vi "Test File Log Provider.vi"() -> (1 "pass?":bool)   [LabVIEW 2019, in "ANODE Tests.lvlib"]
uses:
  ANODE Tests.lvlib
  ANODE/Utility API/Log Service/public/level.ctl
  34bea0a4-f80a-4efe-aaf4-9db1f3a8a041.vi
  4e885d52-342e-4d6f-86c2-bbc79adb3db9.vi
  901ffbec-7f76-4fda-a8b3-ab898965128c.vi
  31a8342b-9139-4bdf-bbc1-bb92f7179d80.vi
  c69379c1-06bc-43e8-abf1-6b6e803fbc34.vi
  7ff86ca6-88c0-4de2-a7d7-e18e6c48d840.vi
  f5e9308b-311a-4c07-9062-c62029aec88d.vi
  cd498dcc-2004-4e95-9cb1-3a88910e2f61.vi
  4bbd3971-874f-4069-8a4a-00f2533dc096.vi
  51edfdbb-9a3d-492a-8a02-2d0f54c6b824.vi
  8f198e5f-b4d0-4ca0-822a-d58fe651c8a2.vi
  ANODE/Util/Timestamp or now.vi
  ANODE/Utility API/File Log Provider/File Log Provider.lvclass
  C:/Users/Nicholas Folse/Documents/workspace/github-tauterra.llc/ANODE/ANODE/Utility API/Log Service/Log Service.lvclass
  ANODE/Utility API/Log Service/Log Service.lvclass
panel:
  out "log file text":string
  out "error out":errorcluster
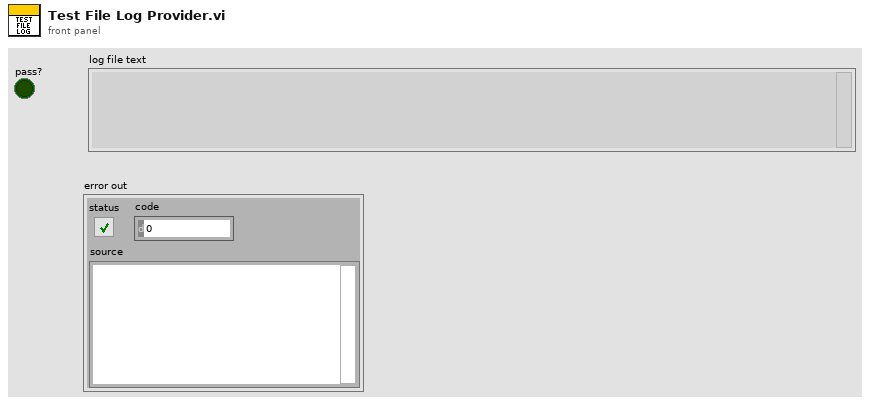
[diagram p1: front panel]
types:
  T1 = typedef "Utility API.lvlib/Log Service.lvclass/level.ctl" = u16
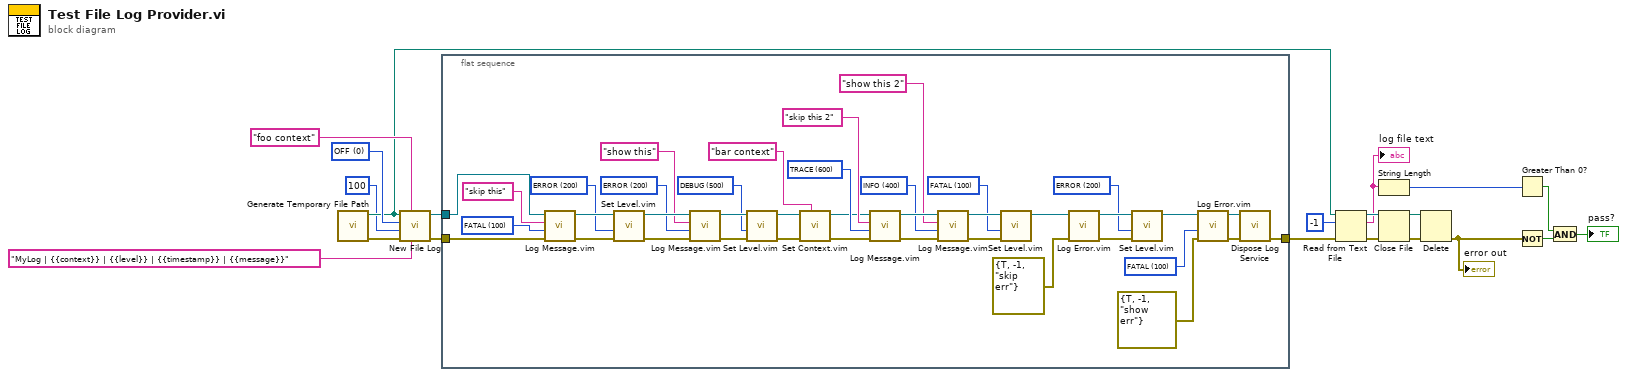
[diagram p0: block diagram]
diagram:
  w19 = T1 0 items=["OFF"=0, "FATAL"=100, "ERROR"=200, "WARN"=300, "INFO"=400, "DEBUG"=500, "TRACE"=600, "ALL"=65535] ("level")
  n1 = call <vilib>:"Generate Temporary File Path.vi"() -> ("error out"=w6:errorcluster, "Unique Temporary File Path"=w16:path)  [unwired: 10 in]
  n2 = call "New File Log.vi"("line format"="MyLog | {{context}} | {{level}} | {{timestamp}} | {{message}}", "context"="foo context", "error in (no error)"=w6, "write timeout (100ms)"=100, "level"=w19, "Path"=w16) -> ("error out"=w17:errorcluster, "File Log Provider out"=w18:refnum<data-value>)  [unwired: 4 in]
  n3 = flat-sequence {
    tunnel: w18 -> [w59]
    tunnel: w17 -> [w51]
    tunnel: [w23] -> w15
    frame #0 {
      w21 = T1 100 items=["OFF"=0, "FATAL"=100, "ERROR"=200, "WARN"=300, "INFO"=400, "DEBUG"=500, "TRACE"=600, "ALL"=65535] ("error level")
      w31 = T1 200 items=["OFF"=0, "FATAL"=100, "ERROR"=200, "WARN"=300, "INFO"=400, "DEBUG"=500, "TRACE"=600, "ALL"=65535] ("level")
      w36 = T1 100 items=["OFF"=0, "FATAL"=100, "ERROR"=200, "WARN"=300, "INFO"=400, "DEBUG"=500, "TRACE"=600, "ALL"=65535] ("level")
      w39 = T1 400 items=["OFF"=0, "FATAL"=100, "ERROR"=200, "WARN"=300, "INFO"=400, "DEBUG"=500, "TRACE"=600, "ALL"=65535] ("level")
      w43 = T1 600 items=["OFF"=0, "FATAL"=100, "ERROR"=200, "WARN"=300, "INFO"=400, "DEBUG"=500, "TRACE"=600, "ALL"=65535] ("level")
      w46 = T1 500 items=["OFF"=0, "FATAL"=100, "ERROR"=200, "WARN"=300, "INFO"=400, "DEBUG"=500, "TRACE"=600, "ALL"=65535] ("level")
      w52 = T1 200 items=["OFF"=0, "FATAL"=100, "ERROR"=200, "WARN"=300, "INFO"=400, "DEBUG"=500, "TRACE"=600, "ALL"=65535] ("level")
      w55 = T1 200 items=["OFF"=0, "FATAL"=100, "ERROR"=200, "WARN"=300, "INFO"=400, "DEBUG"=500, "TRACE"=600, "ALL"=65535] ("level")
      w58 = T1 100 items=["OFF"=0, "FATAL"=100, "ERROR"=200, "WARN"=300, "INFO"=400, "DEBUG"=500, "TRACE"=600, "ALL"=65535] ("level")
      n4 = call "Log Message.vim"("error in (no error)"=w51, "level"=w58, "message"="skip this", "Log Service in"=w59) -> ("error out"=w50:errorcluster, "Log Service out"=w56:refnum<data-value>)  [unwired: 6 in]
      n5 = call "Set Level.vim"("error in (no error)"=w50, "level"=w55, "Log Service in"=w56) -> ("error out"=w49:errorcluster, "Log Service out"=w54:refnum<data-value>)  [unwired: 7 in]
      n6 = call "Log Message.vim"("error in (no error)"=w49, "level"=w52, "message"="show this", "Log Service in"=w54) -> ("error out"=w47:errorcluster, "Log Service out"=w48:refnum<data-value>)  [unwired: 6 in]
      n7 = call "Set Level.vim"("error in (no error)"=w47, "level"=w46, "Log Service in"=w48) -> ("error out"=w27:errorcluster, "Log Service out"=w45:refnum<data-value>)  [unwired: 7 in]
      n8 = call "Set Context.vim"("context"="bar context", "error in (no error)"=w27, "Log Service in"=w45) -> ("error out"=w26:errorcluster, "Log Service out"=w28:refnum<data-value>)  [unwired: 7 in]
      n9 = call "Log Message.vim"("error in (no error)"=w26, "level"=w43, "message"="skip this 2", "Log Service in"=w28) -> ("error out"=w41:errorcluster, "Log Service out"=w42:refnum<data-value>)  [unwired: 6 in]
      n10 = call "Log Message.vim"("error in (no error)"=w41, "level"=w39, "message"="show this 2", "Log Service in"=w42) -> ("error out"=w38:errorcluster, "Log Service out"=w37:refnum<data-value>)  [unwired: 6 in]
      n11 = call "Set Level.vim"("error in (no error)"=w38, "level"=w36, "Log Service in"=w37) -> ("Log Service out"=w35:refnum<data-value>)  [unwired: 7 in, 1 out]
      n12 = call "Log Error.vim"("error in (no error)"=errorcluster {"status"=TRUE, "code"=-1, "source"="skip err"}, "Log Service in"=w35) -> ("error out"=w32:errorcluster, "Log Service out"=w33:refnum<data-value>)  [unwired: 8 in]
      n13 = call "Set Level.vim"("error in (no error)"=w32, "level"=w31, "Log Service in"=w33) -> ("Log Service out"=w30:refnum<data-value>)  [unwired: 7 in, 1 out]
      n14 = call "Log Error.vim"("error in (no error)"=errorcluster {"status"=TRUE, "code"=-1, "source"="show err"}, "error level"=w21, "Log Service in"=w30) -> ("error out"=w22:errorcluster, "Log Service out"=w24:refnum<data-value>)  [unwired: 7 in]
      n15 = call "Dispose Log Service.vi"("error in (no error)"=w22, "Log Service in"=w24) -> ("error out"=w23:errorcluster)  [unwired: 9 in]
    }
  }
  n16 = Read from Text File(file (use dialog)=w16, count=-1, error in=w15) -> (refnum out=w12:refnum<file>, text=w5:string, error out=w13:errorcluster)  [unwired: 1 in, 1 out]
  "log file text" <- w5
  n17 = String Length(string=w5) -> (length=w4:i32)
  n18 = Close File(refnum=w12, error in=w13) -> (path=w11:path, error out=w10:errorcluster)
  n19 = Delete(path (use dialog)=w11, error in=w10) -> (error out=w9:errorcluster)  [unwired: 3 in, 2 out]
  "error out" <- w9
  n20 = Greater Than 0?(x=w4) -> (x > 0?=w2:bool)
  n21 = Not(x=w9) -> (.not. x?=w8:bool)
  n22 = And(x=w2, y=w8) -> (x .and. y?=→"pass?":bool)
